vi "CloseCVandTF.vi"(11 "TFinfo In":T1) -> (3 "TFinfo out":T1)   [LabVIEW 2020]
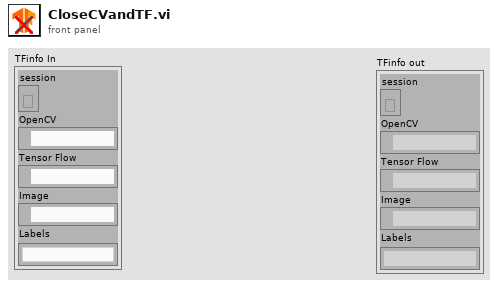
[diagram p1: front panel]
types:
  T1 = cluster{"session":refnum<k35>, "OpenCV":path, "Tensor Flow":path, "Image":path, "Labels":string}
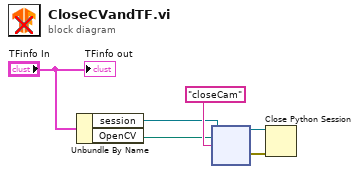
[diagram p0: block diagram]
diagram:
  n1 = Unbundle By Name("TFinfo In") -> ("session"=w3:refnum<k35>, "OpenCV"=w2:path)
  n2 = node(w3, w2, "closeCam" ("function name")) -> (w5:refnum<k35>, w6:errorcluster)  [unwired: 3 in, 2 out]
  n3 = Close Python Session(session in=w5, error in=w6) -> ()  [unwired: 1 out]
  "TFinfo out" <- "TFinfo In"
